vi "FindAdjacentSWFolders.vi"() -> (3 "Array":path[](array[path]))   [LabVIEW 2015]
uses:
  Globals/Constants_global.vi
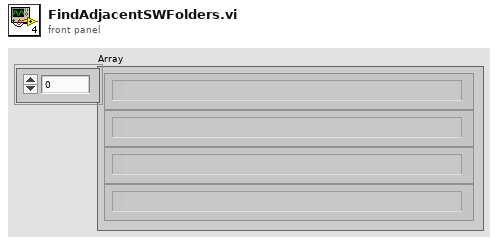
[diagram p1: front panel]
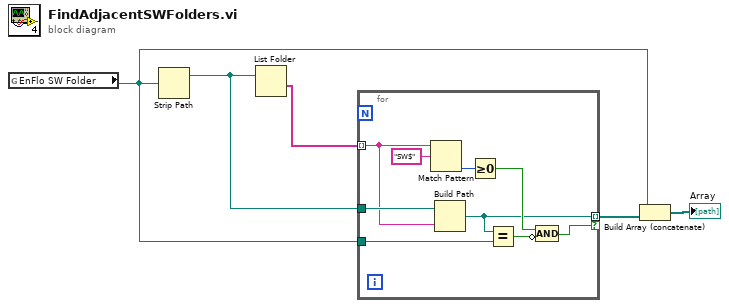
[diagram p0: block diagram]
diagram:
  n1 = global read "Constants_global.vi" "EnFlo SW Folder"() -> (w1:path)
  n2 = Strip Path(path=w1) -> (stripped path=w4:path)  [unwired: 1 out]
  n3 = List Folder(path=w4) -> (folder names=w5:string[])  [unwired: 3 in, 3 out]
  n4 = for {
    tunnel: w5 -> [w12] mode=indexing
    tunnel: w4 -> [w13]
    tunnel: [w9] -> w3 mode=indexing if=w7
    tunnel: w1 -> [w8]
    n5 = Match Pattern(string=w12, regular expression="SW$") -> (offset past match=w11:i32)  [unwired: 1 in, 3 out]
    n6 = Build Path(base path=w13, name or relative path=w12) -> (appended path=w9:path)
    n7 = Greater Or Equal To 0?(x=w11) -> (x >= 0?=w10:bool)
    n8 = Equal?(x=w9, y=w8) -> (x = y?=w6:bool)
    n9 = Compound Arithmetic op=AND(w10, invert w6) -> (w7:bool)
  }
  n10 = Build Array (concatenate)(w1, w3) -> (→"Array":path[])
